vi "Update All Values.vi"(8 "error in (no error)":errorcluster, 10 "Values":refnum<class "Type.lvclass">[](array[class]), 11 "NewEntityTemplate in":refnum<class "MoarDemo.lvclass">) -> (0 "error out":errorcluster, 3 "NewEntityTemplate out":refnum<class "MoarDemo.lvclass">)   [LabVIEW 2020, in "tests.lvlib" / "MoarDemo.lvclass"]
uses:
  MoarDemo.lvclass
  MoarDemo.lvclass/MoarDemo.ctl
  <vilib>/IlluminatedG/IG Conditum Base/Conditum/Columns/Boolean/Boolean.lvclass
  <vilib>/IlluminatedG/IG Conditum Base/Conditum/Columns/Double/Double.lvclass
  <vilib>/IlluminatedG/IG Conditum Base/Conditum/Columns/String/String.lvclass
  <vilib>/IlluminatedG/IG Conditum Base/Conditum/Columns/Type/Type.lvclass
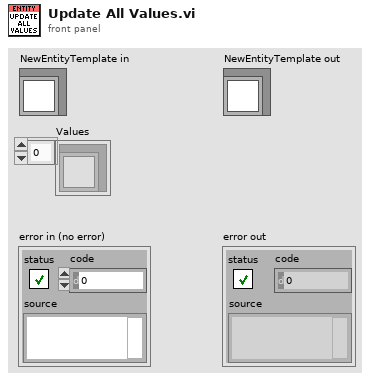
[diagram p1: front panel]
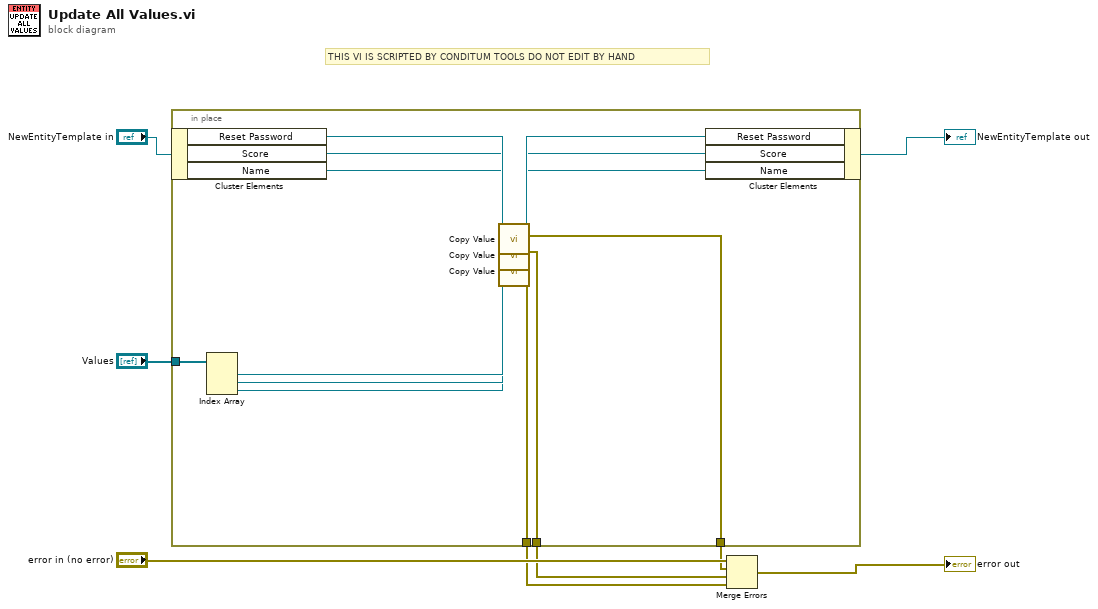
[diagram p0: block diagram]
diagram:
  # "THIS VI IS SCRIPTED BY CONDITUM TOOLS DO NOT EDIT BY HAND"
  n1 = in-place {
    in-place-border: "Values" -> [w21]
    in-place-border: [w20] -> w3
    in-place-border: [w16] -> w2
    in-place-border: [w12] -> w1
    n2 = in-place-cluster #1("NewEntityTemplate in") -> ("Reset Password"=w18:refnum<class "Boolean.lvclass">, "Score"=w14:refnum<class "Double.lvclass">, "Name"=w10:refnum<class "String.lvclass">)
    n3 = Index Array(array=w21) -> (element #1=w17:refnum<class "Type.lvclass">, element #2=w13:refnum<class "Type.lvclass">, element #3=w9:refnum<class "Type.lvclass">)  [unwired: 3 in]
    n4 = call-dynamic "Copy Value.vi"("From"=w17, "Boolean in"=w18) -> ("error out"=w20:errorcluster, "Boolean out"=w19:refnum<class "Boolean.lvclass">)  [unwired: 8 in]
    n5 = call-dynamic "Copy Value.vi"("From"=w13, "Double in"=w14) -> ("error out"=w16:errorcluster, "Double out"=w15:refnum<class "Double.lvclass">)  [unwired: 8 in]
    n6 = call-dynamic "Copy Value.vi"("From"=w9, "String in"=w10) -> ("error out"=w12:errorcluster, "String out"=w11:refnum<class "String.lvclass">)  [unwired: 8 in]
    n7 = in-place-cluster #1("Reset Password"=w19, "Score"=w15, "Name"=w11) -> (→"NewEntityTemplate out":refnum<class "MoarDemo.lvclass">)
  }
  n8 = Merge Errors("error in (no error)", w3, w2, w1) -> (→"error out":errorcluster)
